vi "Main Loop.vi"(8 "Error In":errorcluster, 11 "Process In":refnum<class "Process.lvclass">) -> (0 "Error Out":errorcluster, 3 "Process Out":refnum<class "Process.lvclass">)   [LabVIEW 2019, in "Process.lvclass"]
uses:
  Process.lvclass
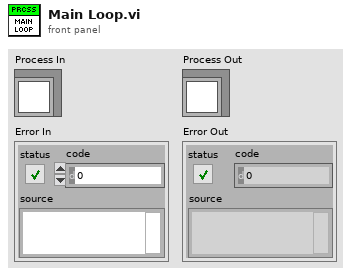
[diagram p1: front panel]
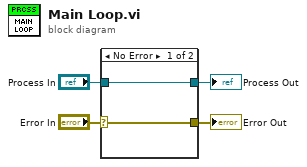
[diagram p0: block diagram]
diagram:
  n1 = case shown="No Error" "Error In" {
    selector: "Error In" -> [w6 w7]
    tunnel: [w6 w7] -> w3
    tunnel: [w5 w8] -> w2
    tunnel: "Process In" -> [w5 w8]
    frame No Error {
    }
    frame Error {
    }
  }
  "Error Out" <- w3
  "Process Out" <- w2
